vi "Trip1_DesiredAngle_DIO_annotated.vi"(0 "Current Angle":dbl format="%#_13g", 2 "X-Position":dbl, 3 "Y-Position":dbl) -> (9 "Zone A":bool, 11 "Zone B":bool, 13 "Commence Mining":bool, 14 "RFM":i32, 15 "RMM":i32, 16 "RRM":i32, 17 "LFM":i32, 18 "LMM":i32, 19 "LRM":i32)   [LabVIEW 2014]
panel:
  out "Desired Angle":dbl
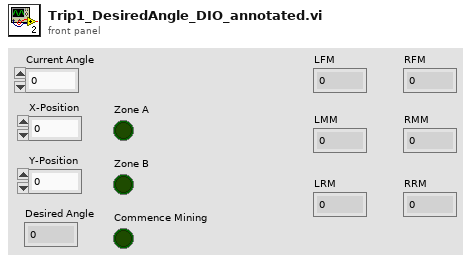
[diagram p1: front panel]
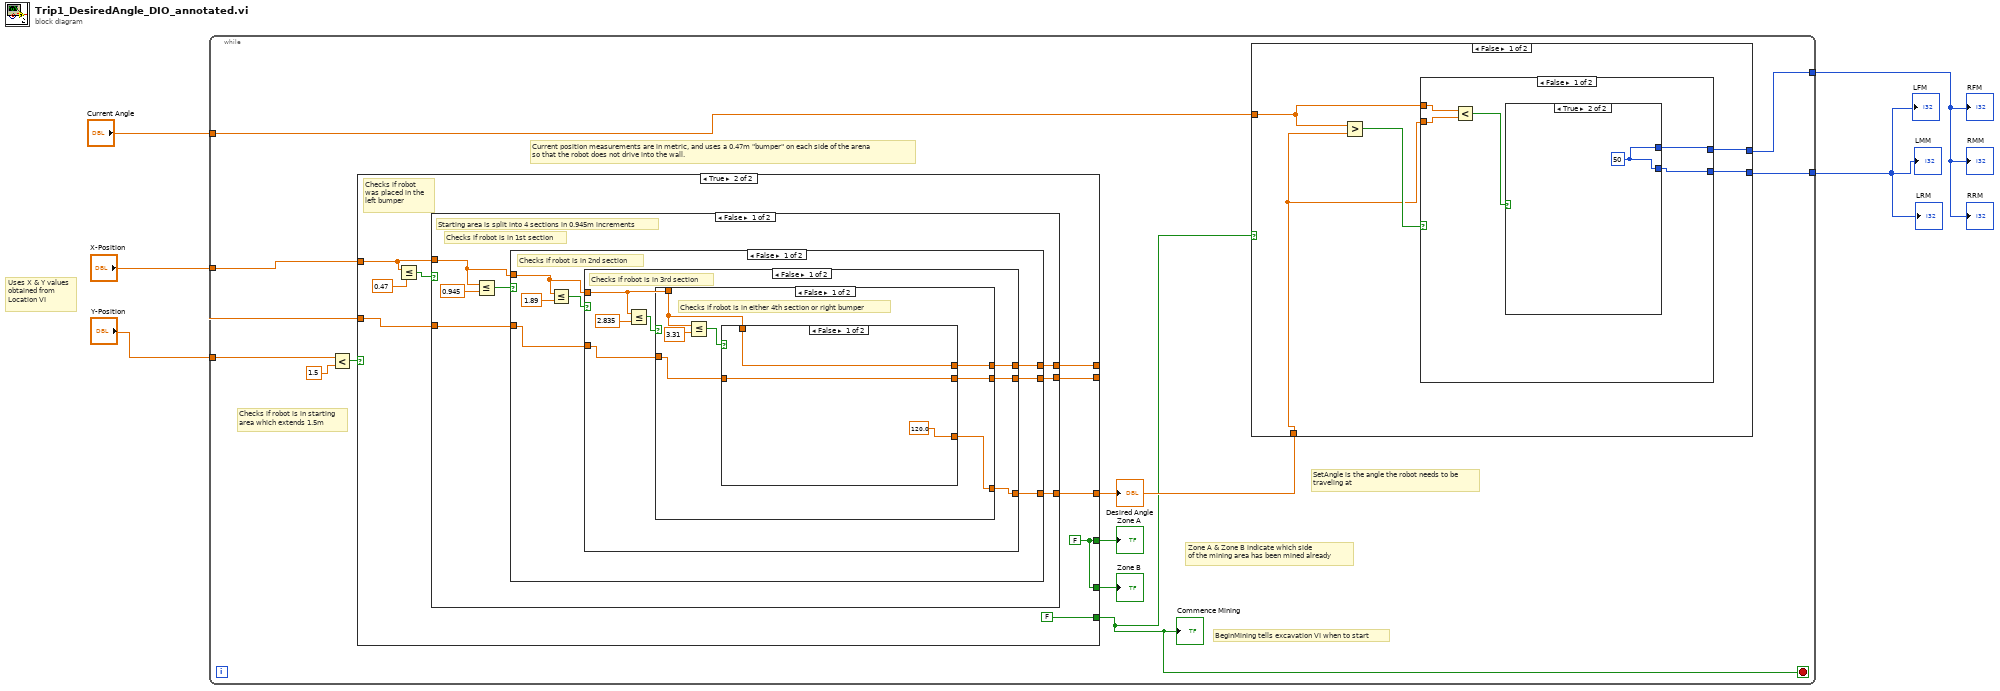
[diagram p0: block diagram]
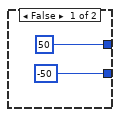
[diagram p2: hidden frame]
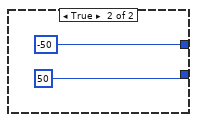
[diagram p3: hidden frame]
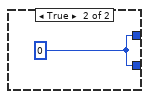
[diagram p4: hidden frame]
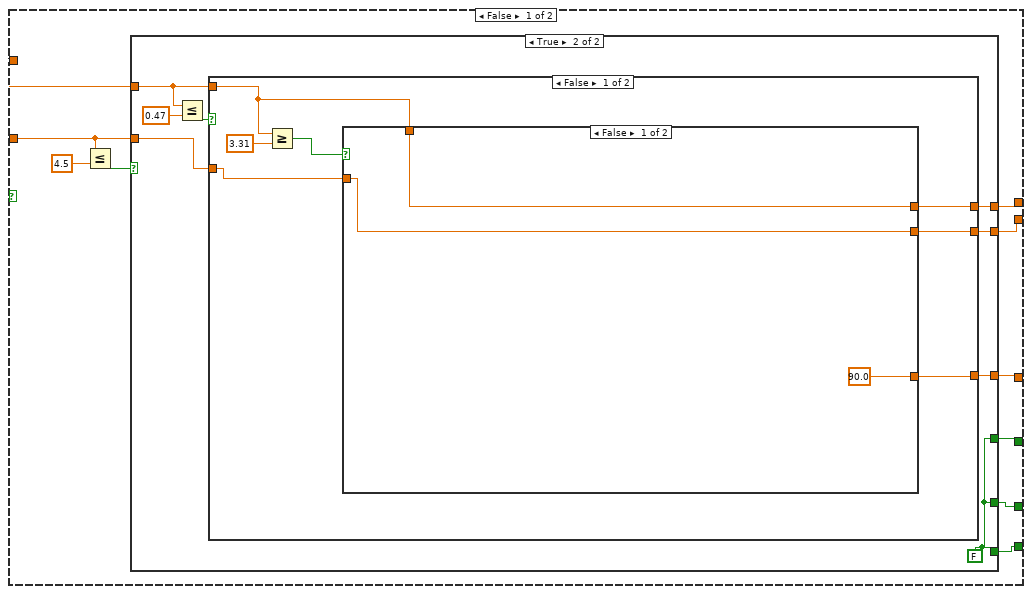
[diagram p5: hidden frame]
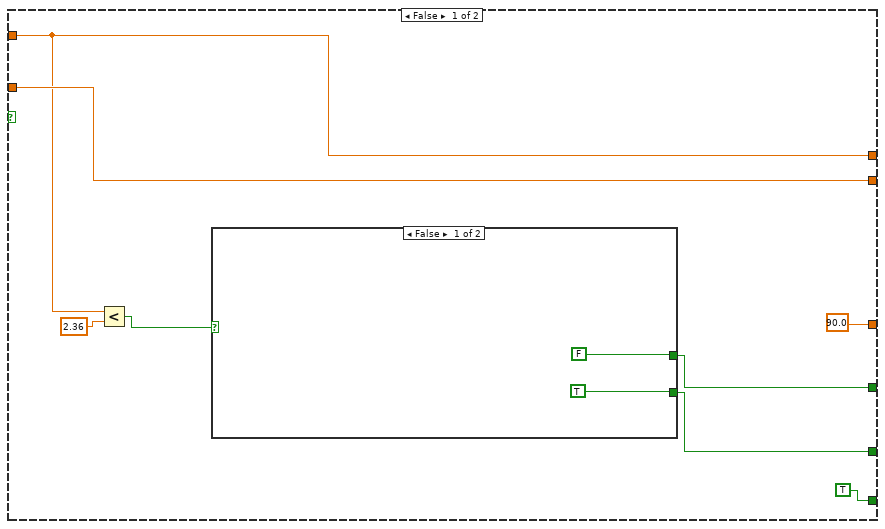
[diagram p6: hidden frame]
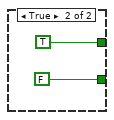
[diagram p7: hidden frame]
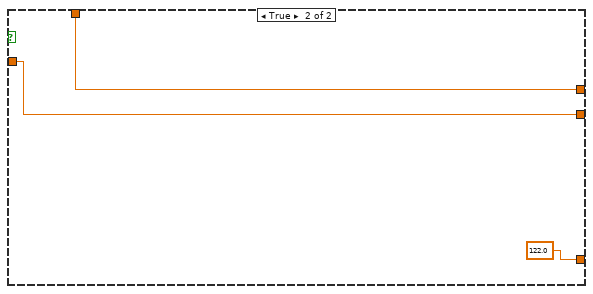
[diagram p8: hidden frame]
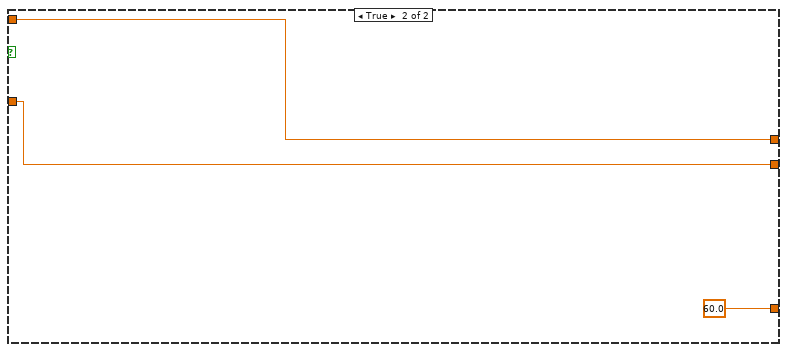
[diagram p9: hidden frame]
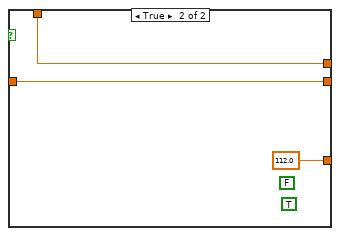
[diagram p10: hidden frame]
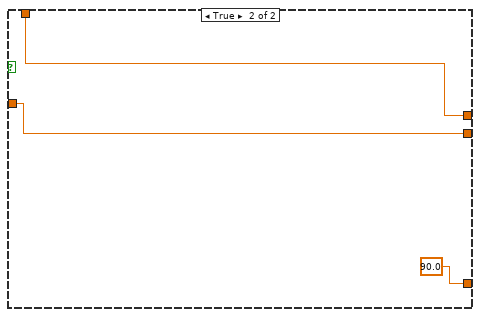
[diagram p11: hidden frame]
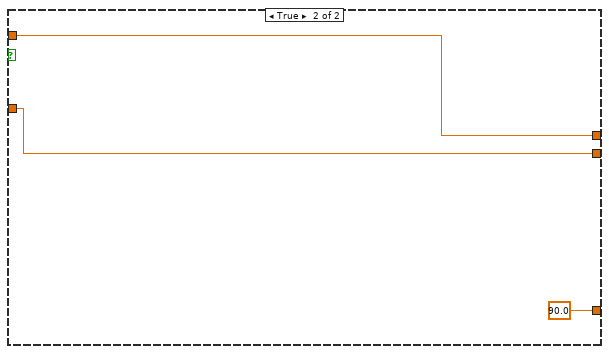
[diagram p12: hidden frame]
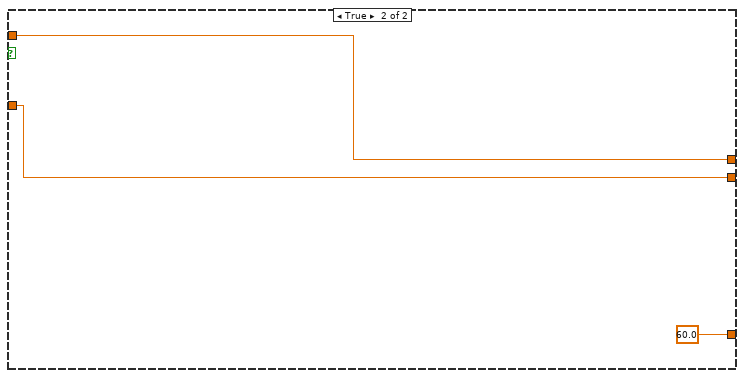
[diagram p13: hidden frame]
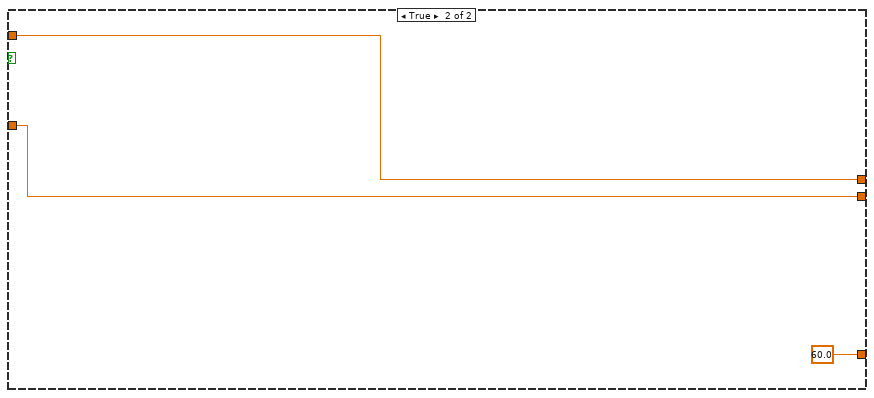
[diagram p14: hidden frame]
diagram:
  # "Uses X & Y values\nobtained from\nLocation VI"
  n1 = while {
    tunnel: "X-Position" -> [w16]
    tunnel: "Y-Position" -> [w15]
    tunnel: "Current Angle" -> [w11]
    tunnel: [w9] -> w2
    tunnel: [w8] -> w1
    stop <- w6 stop-if-true
    # "SetAngle is the angle the robot needs to be\ntraveling at"
    # "Zone A & Zone B indicate which side \nof the mining area has been mined already"
    # "BeginMining tells excavation VI when to start"
    # "Checks if robot is in starting\narea which extends 1.5m"
    # "Current position measurements are in metric, and uses a 0.47m \"bumper\" on each side of the arena\nso that the robot does not drive into the wall."
    n2 = Less?(x=w15, y=1.5) -> (x < y?=w14:bool)
    n3 = case shown="True" w14 {
      tunnel: [w42 w87] -> w10
      tunnel: [w34 w79] -> w13
      tunnel: [w33 w79] -> w12
      tunnel: w16 -> [w41 w85]
      tunnel: [w36 w83] -> _
      tunnel: w15 -> [w38 w82]
      tunnel: [w37 w81] -> _
      tunnel: [w35 FALSE] -> w6
      frame False {
        n4 = Less Or Equal?(x=w38, y=4.5) -> (x <= y?=w39:bool)
        n5 = case shown="True" w39 {
          tunnel: [90.0 w60] -> w42
          tunnel: w41 -> [w47 w59]
          tunnel: w38 -> [w49 w58]
          tunnel: [w49 w57] -> w37
          tunnel: [w47 w56] -> w36
          tunnel: [TRUE w55] -> w35
          tunnel: [w44 w55] -> w34
          tunnel: [w43 w55] -> w33
          frame False {
            n6 = Less?(x=w47, y=2.36) -> (x < y?=w45:bool)
            n7 = case shown="False" w45 {
              tunnel: [FALSE TRUE] -> w44
              tunnel: [TRUE FALSE] -> w43
              frame False {
              }
              frame True {
              }
            }
          }
          frame True {
            w55 = FALSE
            n8 = Less Or Equal?(x=w59, y=0.47) -> (x <= y?=w61:bool)
            n9 = case shown="False" w61 {
              tunnel: [w67 60.0] -> w60
              tunnel: w59 -> [w66 w77]
              tunnel: w58 -> [w65 w76]
              tunnel: [w64 w76] -> w57
              tunnel: [w63 w77] -> w56
              frame False {
                n10 = Greater Or Equal?(x=w66, y=3.31) -> (x >= y?=w68:bool)
                n11 = case shown="False" w68 {
                  tunnel: [90.0 122.0] -> w67
                  tunnel: w66 -> [w70 w74]
                  tunnel: w65 -> [w71 w73]
                  tunnel: [w71 w73] -> w64
                  tunnel: [w70 w74] -> w63
                  frame False {
                  }
                  frame True {
                  }
                }
              }
              frame True {
              }
            }
          }
        }
      }
      frame True {
        w79 = FALSE
        # "Checks if robot\nwas placed in the \nleft bumper"
        n12 = Less Or Equal?(x=w85, y=0.47) -> (x <= y?=w84:bool)
        n13 = case shown="False" w84 {
          tunnel: w85 -> [w92 w132]
          tunnel: [w91 60.0] -> w87
          tunnel: [w90 w132] -> w83
          tunnel: w82 -> [w89 w131]
          tunnel: [w88 w131] -> w81
          frame False {
            # "Checks if robot is in 1st section"
            # "Starting area is split into 4 sections in 0.945m increments"
            n14 = Less Or Equal?(x=w92, y=0.945) -> (x <= y?=w94:bool)
            n15 = case shown="False" w94 {
              tunnel: w92 -> [w99 w129]
              tunnel: [w98 60.0] -> w91
              tunnel: [w97 w129] -> w90
              tunnel: w89 -> [w96 w128]
              tunnel: [w95 w128] -> w88
              frame False {
                # "Checks if robot is in 2nd section"
                n16 = Less Or Equal?(x=w99, y=1.89) -> (x <= y?=w100:bool)
                n17 = case shown="False" w100 {
                  tunnel: w99 -> [w106 w126]
                  tunnel: [w105 90.0] -> w98
                  tunnel: [w104 w126] -> w97
                  tunnel: w96 -> [w103 w125]
                  tunnel: [w102 w125] -> w95
                  frame False {
                    # "Checks if robot is in 3rd section"
                    n18 = Less Or Equal?(x=w106, y=2.835) -> (x <= y?=w107:bool)
                    n19 = case shown="False" w107 {
                      tunnel: w106 -> [w113 w123]
                      tunnel: [w112 90.0] -> w105
                      tunnel: [w111 w123] -> w104
                      tunnel: w103 -> [w110 w122]
                      tunnel: [w109 w122] -> w102
                      frame False {
                        # "Checks if robot is in either 4th section or right bumper"
                        n20 = Less Or Equal?(x=w113, y=3.31) -> (x <= y?=w114:bool)
                        n21 = case shown="False" w114 {
                          tunnel: w113 -> [w117 w120]
                          tunnel: [120.0 112.0] -> w112
                          tunnel: [w117 w120] -> w111
                          tunnel: w110 -> [w116 w119]
                          tunnel: [w116 w119] -> w109
                          frame False {
                          }
                          frame True {
                            (unwired) TRUE
                            (unwired) FALSE
                          }
                        }
                      }
                      frame True {
                      }
                    }
                  }
                  frame True {
                  }
                }
              }
              frame True {
              }
            }
          }
          frame True {
          }
        }
      }
    }
    "Desired Angle" <- w10
    "Zone A" <- w13
    "Zone B" <- w12
    "Commence Mining" <- w6
    n22 = case shown="False" w6 {
      tunnel: w11 -> [w20 _]
      tunnel: w10 -> [w19 _]
      tunnel: [w17 w32] -> w9
      tunnel: [w18 w32] -> w8
      frame False {
        n23 = Greater?(x=w20, y=w19) -> (0:w21:bool)
        n24 = case shown="False" w21 {
          tunnel: w20 -> [w26 _]
          tunnel: w19 -> [w25 _]
          tunnel: [w23 -50] -> w18
          tunnel: [w22 50] -> w17
          frame False {
            n25 = Less?(x=w26, y=w25) -> (x < y?=w24:bool)
            n26 = case shown="True" w24 {
              tunnel: [50 w29] -> w23
              tunnel: [-50 w29] -> w22
              frame False {
              }
              frame True {
                w29 = 50
              }
            }
          }
          frame True {
          }
        }
      }
      frame True {
        w32 = 0
      }
    }
  }
  "LFM" <- w2
  "LMM" <- w2
  "LRM" <- w2
  "RFM" <- w1
  "RMM" <- w1
  "RRM" <- w1
